vi "liquid flow formulas (SubVI).vi"(4 "LFP Offset 4":dbl, 7 "LFP Offset in":dbl, 9 "LFP Offset 1":dbl, 11 "LFP Offset 3":dbl, 12 "LFB Offset":dbl, 13 "unsigned byte array":u8[](array[numeric])) -> (10 "Numeric":dbl, 14 "Numeric 5":dbl, 15 "Numeric 4":dbl, 16 "Numeric 3":dbl, 17 "Numeric 2":dbl)   [LabVIEW 2016]
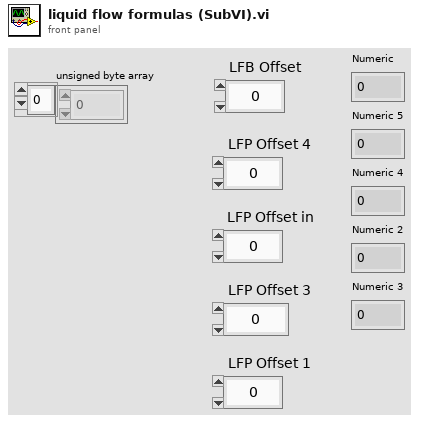
[diagram p1: front panel]
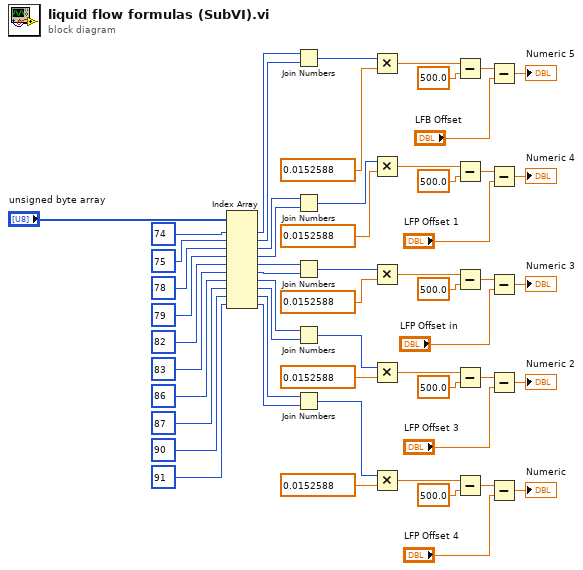
[diagram p0: block diagram]
diagram:
  n1 = Index Array(array="unsigned byte array", index #1=74 ("index"), index #2=75 ("index"), index #3=78 ("index"), index #4=79 ("index"), index #5=82 ("index"), index #6=83 ("index"), index #7=86 ("index"), index #8=87 ("index"), index #9=90 ("index"), index #10=91 ("index")) -> (element #1=w17:u8, element #2=w16:u8, element #3=w15:u8, element #4=w14:u8, element #5=w11:u8, element #6=w10:u8, element #7=w6:u8, element #8=w5:u8, element #9=w2:u8, element #10=w1:u8)
  n2 = Join Numbers(hi=w17, lo=w16) -> ((hi.lo)=w22:u16)
  n3 = Join Numbers(hi=w15, lo=w14) -> ((hi.lo)=w29:u16)
  n4 = Join Numbers(hi=w11, lo=w10) -> ((hi.lo)=w33:u16)
  n5 = Join Numbers(hi=w6, lo=w5) -> ((hi.lo)=w37:u16)
  n6 = Join Numbers(hi=w2, lo=w1) -> ((hi.lo)=w41:u16)
  n7 = Multiply(x=w22, y=0.0152588) -> (x*y=w24:dbl)
  n8 = Multiply(x=w29, y=0.0152588) -> (x*y=w27:dbl)
  n9 = Multiply(x=w33, y=0.0152588) -> (x*y=w31:dbl)
  n10 = Multiply(x=w37, y=0.0152588) -> (x*y=w35:dbl)
  n11 = Multiply(x=w41, y=0.0152588) -> (x*y=w39:dbl)
  n12 = Subtract(x=w24, y=500.0) -> (x-y=w42:dbl)
  n13 = Subtract(x=w27, y=500.0) -> (x-y=w46:dbl)
  n14 = Subtract(x=w31, y=500.0) -> (x-y=w48:dbl)
  n15 = Subtract(x=w35, y=500.0) -> (x-y=w51:dbl)
  n16 = Subtract(x=w39, y=500.0) -> (x-y=w54:dbl)
  n17 = Subtract(x=w42, y="LFB Offset") -> (x-y=→"Numeric 5":dbl)
  n18 = Subtract(x=w46, y="LFP Offset 1") -> (x-y=→"Numeric 4":dbl)
  n19 = Subtract(x=w48, y="LFP Offset in") -> (x-y=→"Numeric 3":dbl)
  n20 = Subtract(x=w51, y="LFP Offset 3") -> (x-y=→"Numeric 2":dbl)
  n21 = Subtract(x=w54, y="LFP Offset 4") -> (x-y=→"Numeric":dbl)
